vi "write freq and power.vi"(4 "leveling":bool=TRUE, 6 "leviling file":path=path "C:/Users/Ouyang Group/Documents/Data/8-26-16/Windfreak plus switches and amp power calibration high res", 7 "Channel":bool=TRUE, 8 "RF On":bool, 9 "p (dbm)":dbl=-9.0, 10 "f (Hz)":dbl=3947917162.722741, 11 "Serial Port Select":refnum<visa-resource-name>="ASRL14::INSTR") -> (2 "COM Error":bool, 3 "Level":bool)   [LabVIEW 2012]
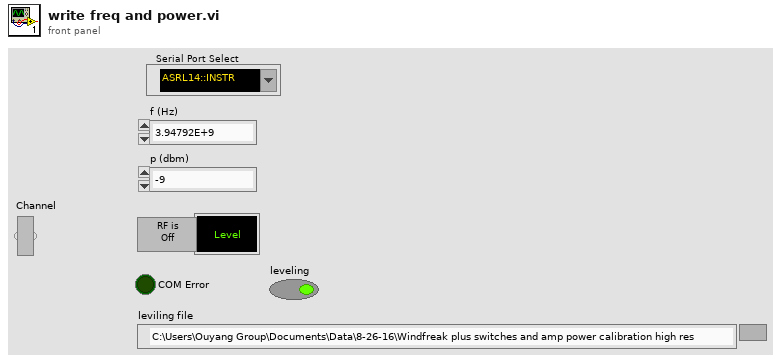
[diagram p1: front panel]
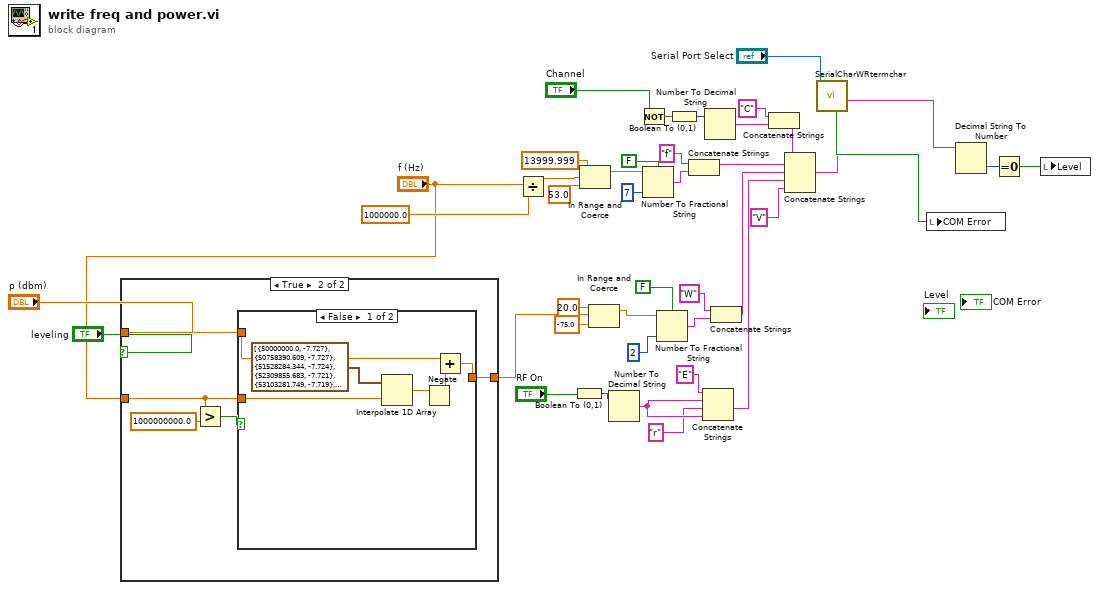
[diagram p0: block diagram]
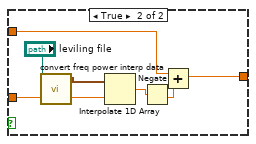
[diagram p3: hidden frame]
diagram:
  n1 = case shown="True" "leveling" {
    tunnel: "p (dbm)" -> [w42 w47]
    tunnel: [w42 w46] -> w7
    tunnel: "f (Hz)" -> [_ w44]
    frame False {
    }
    frame True {
      n2 = Greater?(x=w44, y=1000000000.0) -> (0:w45:bool)
      n3 = case shown="False" w45 {
        tunnel: w44 -> [w51 w58]
        tunnel: w47 -> [w49 w57]
        tunnel: [w48 w56] -> w46
        frame False {
          n4 = Interpolate 1D Array(1:w51, 2:cluster{dbl, dbl}[] [{50000000.0, -7.727}, {50758390.609, -7.727}, {51528284.344, -7.724}, {52309855.683, -7.721}, {53103281.749, -7.719}, {53908742.353, -7.717}, {54726420.031, -7.713}, {55556500.091, -7.707}, {56399170.65, -7.705}, {57254622.678, -7.704}, {58123050.041, -7.702}, {59004649.547, -7.697}, {59899620.989, -7.692}, {60808167.19, -7.69}, {61730494.048, -7.69}, {62666810.588, -7.693}, {63617329.0, -7.696}, {64582264.698, -7.699}, {65561836.359, -7.703}, {66556265.979, -7.704}, {67565778.921, -7.705}, {68590603.965, -7.708}, {69630973.363, -7.709}, {70687122.889, -7.712}, {71759291.892, -7.711}, {72847723.354, -7.714}, {73952663.939, -7.719}, {75074364.056, -7.721}, {76213077.909, -7.722}, {77369063.56, -7.719}, {78542582.985, -7.72}, {79733902.131, -7.722}, {80943290.983, -7.723}, {82171023.618, -7.722}, {83417378.271, -7.722}, {84682637.396, -7.723}, {85967087.735, -7.722}, {87271020.376, -7.72}, {88594730.821, -7.72}, {89938519.058, -7.719}, {91302689.623, -7.721}, {92687551.67, -7.719}, {94093419.045, -7.716}, {95520610.353, -7.713}, {96969449.03, -7.712}, {98440263.419, -7.712}, {99933386.846, -7.713}, {101449157.688, -7.711}, {102987919.457, -7.711}, {104550020.876, -7.71}, {106135815.956, -7.714}, {107745664.078, -7.718}, {109379930.073, -7.723}, {111038984.309, -7.729}, {112723202.767, -7.734}, {114432967.135, -7.742}, {116168664.887, -7.752}, {117930689.377, -7.764}, {119719439.924, -7.778}, {121535321.903, -7.791}, {123378746.838, -7.806}, {125250132.497, -7.818}, {127149902.982, -7.832}, {129078488.829, -7.846}, {131036327.104, -7.86}, {133023861.502, -7.875}, {135041542.448, -7.885}, {137089827.2, -7.896}, {139169179.951, -7.905}, {141280071.933, -7.915}, {143422981.529, -7.923}, {145598394.374, -7.933}, {147806803.474, -7.942}, {150048709.307, -7.951}, {152324619.948, -7.961}, {154635051.173, -7.966}, {156980526.585, -7.971}, {159361577.728, -7.974}, {161778744.208, -7.98}, {164232573.814, -7.986}, {166723622.647, -7.99}, {169252455.241, -7.993}, {171819644.693, -7.997}, {174425772.792, -8.008}, {177071430.153, -8.015}, {179757216.347, -8.027}, {182483740.043, -8.031}, {185251619.137, -8.042}, {188061480.902, -8.045}, {190913962.122, -8.052}, {193809709.242, -8.067}, {196749378.51, -8.095}, {199733636.129, -8.136}, {202763158.407, -8.183}, {205838631.911, -8.231}, {208960753.619, -8.277}, {212130231.082, -8.319}, {215347782.584, -8.359}, {218614137.303, -8.406}, {221930035.478, -8.46}, {225296228.572, -8.517}, {228713479.452, -8.567}, {232182562.551, -8.604}, {235704264.05, -8.632}, {239279382.057, -8.653}, {242908726.782, -8.683}, {246593120.726, -8.713}, {250333398.866, -8.731}, {254130408.842, -8.746}, {257985011.152, -8.765}, {261898079.346, -8.804}, {265870500.223, -8.841}, {269903174.034, -8.865}, {273997014.684, -8.879}, {278152949.94, -8.888}, {282371921.641, -8.905}, {286654885.913, -8.935}, {291002813.382, -8.96}, {295416689.399, -8.977}, {299897514.258, -8.973}, {304446303.427, -8.971}, {309064087.776, -8.976}, {313751913.81, -8.988}, {318510843.909, -8.988}, {323341956.566, -8.971}, {328246346.633, -8.947}, {333225125.566, -8.921}, {338279421.684, -8.909}, {343410380.416, -8.918}, {348619164.566, -8.95}, {353906954.576, -8.982}, {359274948.791, -9.004}, {364724363.734, -9.02}, {370256434.38, -9.037}, {375872414.435, -9.048}, {381573576.62, -9.043}, {387361212.962, -9.037}, {393236635.085, -9.028}, {399201174.508, -9.018}, {405256182.944, -8.977}, {411403032.611, -8.91}, {417643116.539, -8.825}, {423977848.888, -8.754}, {430408665.267, -8.707}, {436937023.062, -8.718}, {443564401.761, -8.787}, {450292303.296, -8.88}, {457122252.377, -8.969}, {464055796.844, -9.032}, {471094508.01, -9.084}, {478239981.026, -9.11}, {485493835.234, -9.134}, {492857714.54, -9.169}, {500333287.785, -9.199}, {507922249.121, -9.245}, {515626318.396, -9.313}, {523447241.548, -9.435}, {531386790.992, -9.56}, {539446766.032, -9.655}, {547628993.259, -9.685}, {555935326.972, -9.668}, {564367649.595, -9.637}, {572927872.103, -9.632}, {581617934.459, -9.69}, {590439806.048, -9.817}, {599395486.128, -9.996}, {608487004.282, -10.149}, {617716420.876, -10.193}, {627085827.527, -10.1}, {636597347.578, -9.915}, {646253136.579, -9.736}, {656055382.774, -9.647}, {666006307.599, -9.672}, {676108166.182, -9.754}, {686363247.858, -9.807}, {696773876.687, -9.778}, {707342411.98, -9.688}, {718071248.83, -9.611}, {728962818.663, -9.595}, {740019589.781, -9.667}, {751244067.926, -9.777}, {762638796.849, -9.854}, {774206358.879, -9.862}, {785949375.517, -9.817}, {797870508.026, -9.804}, {809972458.034, -9.882}, {822257968.147, -10.045}, {834729822.57, -10.214}, {847390847.738, -10.287}, {860243912.958, -10.298}, {873291931.057, -10.345}, {886537859.043, -10.509}, {899984698.778, -10.574}, {913635497.652, -10.699}, {927493349.279, -10.743}, {941561394.198, -10.672}, {955842820.579, -10.575}, {970340864.953, -10.477}, {985058812.941, -10.388}, {1000000000.0, -10.309}] ("Array")) -> (0:w52:dbl)
          n5 = Negate(x=w52) -> (-x=w50:dbl)
          n6 = Add(x=w49, y=w50) -> (x+y=w48:dbl)
        }
        frame True {
          n7 = call "convert freq power interp data.vi"("file path (dialog if empty)"="leviling file") -> ("Array"=w59:cluster{dbl, dbl}[])  [unwired: 10 in]
          n8 = Interpolate 1D Array(1:w58, 2:w59) -> (0:w55:dbl)
          n9 = Negate(x=w55) -> (-x=w54:dbl)
          n10 = Add(x=w57, y=w54) -> (x+y=w56:dbl)
        }
      }
    }
  }
  n11 = Divide(x="f (Hz)", y=1000000.0) -> (x/y=w12:dbl)
  n12 = Boolean To (0,1)(Boolean="RF On") -> (0, 1=w18:i16)
  n13 = In Range and Coerce(upper limit=13999.999, x=w12, lower limit=53.0) -> (coerced(x)=w32:dbl)  [unwired: 1 out]
  n14 = In Range and Coerce(upper limit=20.0, x=w7, lower limit=-75.0) -> (coerced(x)=w23:dbl)  [unwired: 1 out]
  n15 = Number To Decimal String(number=w18) -> (decimal integer string=w17:string)  [unwired: 1 in]
  n16 = Not(x="Channel") -> (.not. x?=w4:bool)
  n17 = Number To Fractional String(use system decimal point (T)=FALSE, number=w32, precision (6)=i16 7) -> (F-format string=w31:string)  [unwired: 1 in]
  n18 = Number To Fractional String(use system decimal point (T)=FALSE, number=w23, precision (6)=i16 2) -> (F-format string=w25:string)  [unwired: 1 in]
  n19 = Boolean To (0,1)(Boolean=w4) -> (0, 1=w6:i16)
  n20 = Concatenate Strings("f" ("element"), w31) -> (w29:string)
  n21 = Concatenate Strings("E" ("element"), w17, "r" ("string"), w17) -> (w14:string)
  n22 = Number To Decimal String(number=w6) -> (decimal integer string=w5:string)  [unwired: 1 in]
  n23 = Concatenate Strings("W" ("string"), w25) -> (w20:string)
  n24 = Concatenate Strings("C" ("element"), w5) -> (w1:string)
  n25 = Concatenate Strings(w1, w29, w20, w14, "V" ("string")) -> (w40:string)
  n26 = call "SerialCharWRtermchar.vi"("VISA resource name"="Serial Port Select", "write buffer"=w40) -> ("error?"=w41:bool, "read buffer"=w37:string)  [unwired: 6 in, 1 out]
  n27 = local write "COM Error"(w41) -> ()
  n28 = Decimal String To Number(string=w37) -> (number=w38:i32)  [unwired: 2 in, 1 out]
  n29 = Equal To 0?(x=w38) -> (x = 0?=w39:bool)
  n30 = local write "Level"(w39) -> ()
